vi "FINAL_PROJECT.vi"() -> ()   [LabVIEW 2014]
panel:
  in  "Blank Button 8":bool caption="Blank Button"
  in  "Blank Button 7":bool caption="Blank Button"
  in  "Blank Button 6":bool caption="Blank Button"
  in  "Blank Button 5":bool caption="Blank Button"
  out "LBV":bool
  out "MBV":bool
  out "HBV":bool
  in  "Blank Button 4":bool caption="Blank Button"
  in  "Blank Button 3":bool caption="Blank Button"
  in  "Blank Button 2":bool caption="Blank Button"
  in  "Blank Button":bool
  out "L":bool
  in  "Air Compressor\nstopped/breakdown":bool
  out "Instrument Air Pressure Gauge (Bar)":dbl(knob) scale=0.0..10.0
  out "H":bool
  out "H":bool
  out "Vibration(mm)":u8(slide) scale=0.0..10.0
  out "GD\n%LEL":u8(slide) scale=0.0..20.0
  out "GD":dbl
  out "Vibration Sensor":dbl
  out "H":bool
  out "High Bank Pressure":u8(slide) scale=0.0..400.0
  out "Medium Bank Pressure":u8(slide) scale=0.0..400.0
  out "Low Bank Pressure":u8(slide) scale=0.0..400.0
  out "Storage Pressure Trend":dbl(graph)
  in  "MB Set-point":dbl
  in  "LB Set-point":dbl
  out "Low Bank Pressure":dbl
  out "MB Trend":dbl(graph) caption="LB Trend"
  out "Medium Bank Pressure":dbl
  out "LB Trend":dbl(graph) caption="MB Trend"
  out "High Bank Pressure":dbl
  out "HB Trend":dbl(graph)
  out "H":bool
  out "L":bool
  in  "Low Stage-3 Temperature (After-Cooler) Set-Point":dbl
  in  "High Stage-3 Temperature (After-Cooler) Set-Point":dbl
  in  "Low Stage-3 Temperature Set-Point":dbl
  in  "High Stage-3 Temperature  Set-Point":dbl
  out "H":bool
  out "L":bool
  in  "Low Stage-3 Pressure  Set-Point":dbl
  in  "High Stage-3 Pressure \nSet-Point":dbl
  out "H":bool
  out "L":bool
  out "3-Stage Pressure":u8(slide) scale=0.0..400.0
  out "3-Stage Temperature (After Cooler)":u8(slide) scale=0.0..250.0
  out "3-Stage Temperature":u8(slide) scale=0.0..250.0
  out "3-Stage Pressure":dbl
  out "3-Stage Temperature (After Cooler)":dbl
  out "3-Stage Temperature":dbl
  out "H":bool
  out "L":bool
  in  "Low Stage-2 Temperature (After-Cooler) Set-Point":dbl
  in  "High Stage-2 Temperature (After-Cooler) Set-Point":dbl
  in  "Low Stage-1 Temperature  Set-Point  2":dbl
  in  "High Stage-2 Temperature  Set-Point":dbl
  out "H":bool
  out "L":bool
  in  "Low Stage-2 Pressure  Set-Point":dbl
  in  "High Stage-2 Pressure          Set-Point":dbl
  out "H":bool
  out "L":bool
  out "2-Stage Pressure":u8(slide) scale=0.0..400.0
  out "2-Stage Temperature (After Cooler)":u8(slide) scale=0.0..250.0
  out "2-Stage Temperature":u8(slide) scale=0.0..250.0
  out "2-Stage Pressure":dbl
  out "2-Stage Temperature (After Cooler)":dbl
  out "2-Stage Temperature":dbl
  in  "Critical Vibration Value":dbl
  in  "Gas Detector %LEL       Set-point":dbl
  out "H":bool
  out "L":bool
  in  "Low Stage-1 Temperature (After-Cooler) Set-Point  2":dbl
  in  "High Stage-1 Temperature (After-Cooler) Set-Point":dbl
  in  "Low Stage-1 Temperature  Set-Point":dbl
  in  "High Stage-1 Temperature  Set-Point":dbl
  out "H":bool
  out "L":bool
  out "MFM Total Kg (Inlet)":dbl format="%#_9g"
  in  "Wire cut":bool
  out "Inlet MFM Total Kg Trend (Kg)":dbl(graph)
  out "Discharge MFM Total Kg Trend (Kg)":dbl(graph)
  out "Inlet MFM Flow Rate Trend (Kg/m2)":dbl(graph)
  out "Discharge MFM Flow Rate Trend (Kg/m2)":dbl(graph)
  out "MFM Flow Rate (Discharge)":dbl
  out "MFM Flow Rate (Inlet)":dbl
  out "MFM Total Kg (Discharge)":dbl format="%#_9g"
  out "Storage Pressure":u8(slide) scale=0.0..400.0
  out "De-pressurizing Diaphram Valve":bool
  out "Suction Valve":bool
  in  "Storage /HB Pressure Set-Point":dbl
  out "CO2 Flooding in Progress":bool
  in  "Fire":bool
  out "Fire Detector-2":bool
  out "Fire Detector-1":bool
  out "ESD":bool
  out "Communication Status":string
  out "Compressor Running Status":string
  in  "Low Stage-1 Pressure  Set-Point":dbl
  in  "High Stage-1 Pressure          Set-Point":dbl
  out "H":bool
  out "L":bool
  out "TT-01":dbl
  out "1-Stage Pressure":u8(slide) scale=0.0..400.0
  out "1-Stage Temperature (After Cooler)":u8(slide) scale=0.0..250.0
  out "1-Stage Temperature":u8(slide) scale=0.0..250.0
  out "PT-11":dbl
  out "1-Stage Temperature (After Cooler)":dbl
  out "TT-11":dbl
  in  "Emergency Shutdown":bool
  out "PT-01":dbl
  out "L":bool
  out "H":bool
  in  "Low Inlet Pressure  Set-Point":dbl
  in  "High Inlet Pressure          Set-Point":dbl
  out "Inlet Temperature":u8(slide) scale=0.0..250.0
  out "Inlet Pressure":u8(slide) scale=0.0..40.0
  # "OPERATING PARAMETERS-PRESSURE (barg)"
  # "Suction MFM"
  # "BV"
  # "Filter"
  # "Cooler"
  # "Suction Valve"
  # "Cooler"
  # "OPERATING PARAMETERS-MASS FLOW"
  # "OPERATING PARAMETERS-TEMPERATURE (degC)"
  # "HBV"
  # "Inlet Stage Operating Parameters"
  # "Stage-I Operating Parameters"
  # "Stage-II Operating Parameters"
  # "Stage-III Operating Parameters"
  # "De-Pressurizing\nDiaphragm\nValve"
  # "OPERATING\nPARAMETERS-VIBRATION\n& GAS LEAK"
  # "MBV"
  # "Cooler"
  # "LBV"
  # "Discharge MFM"
  # "CV"
  # "CONFIGURE SET-POINTS"
  # "FIRE SUPPRESSION SAFETY INTERLOCK"
  # "OPERATING PRESSURE TREND"
  # "OPERATING MASS FLOW TREND"
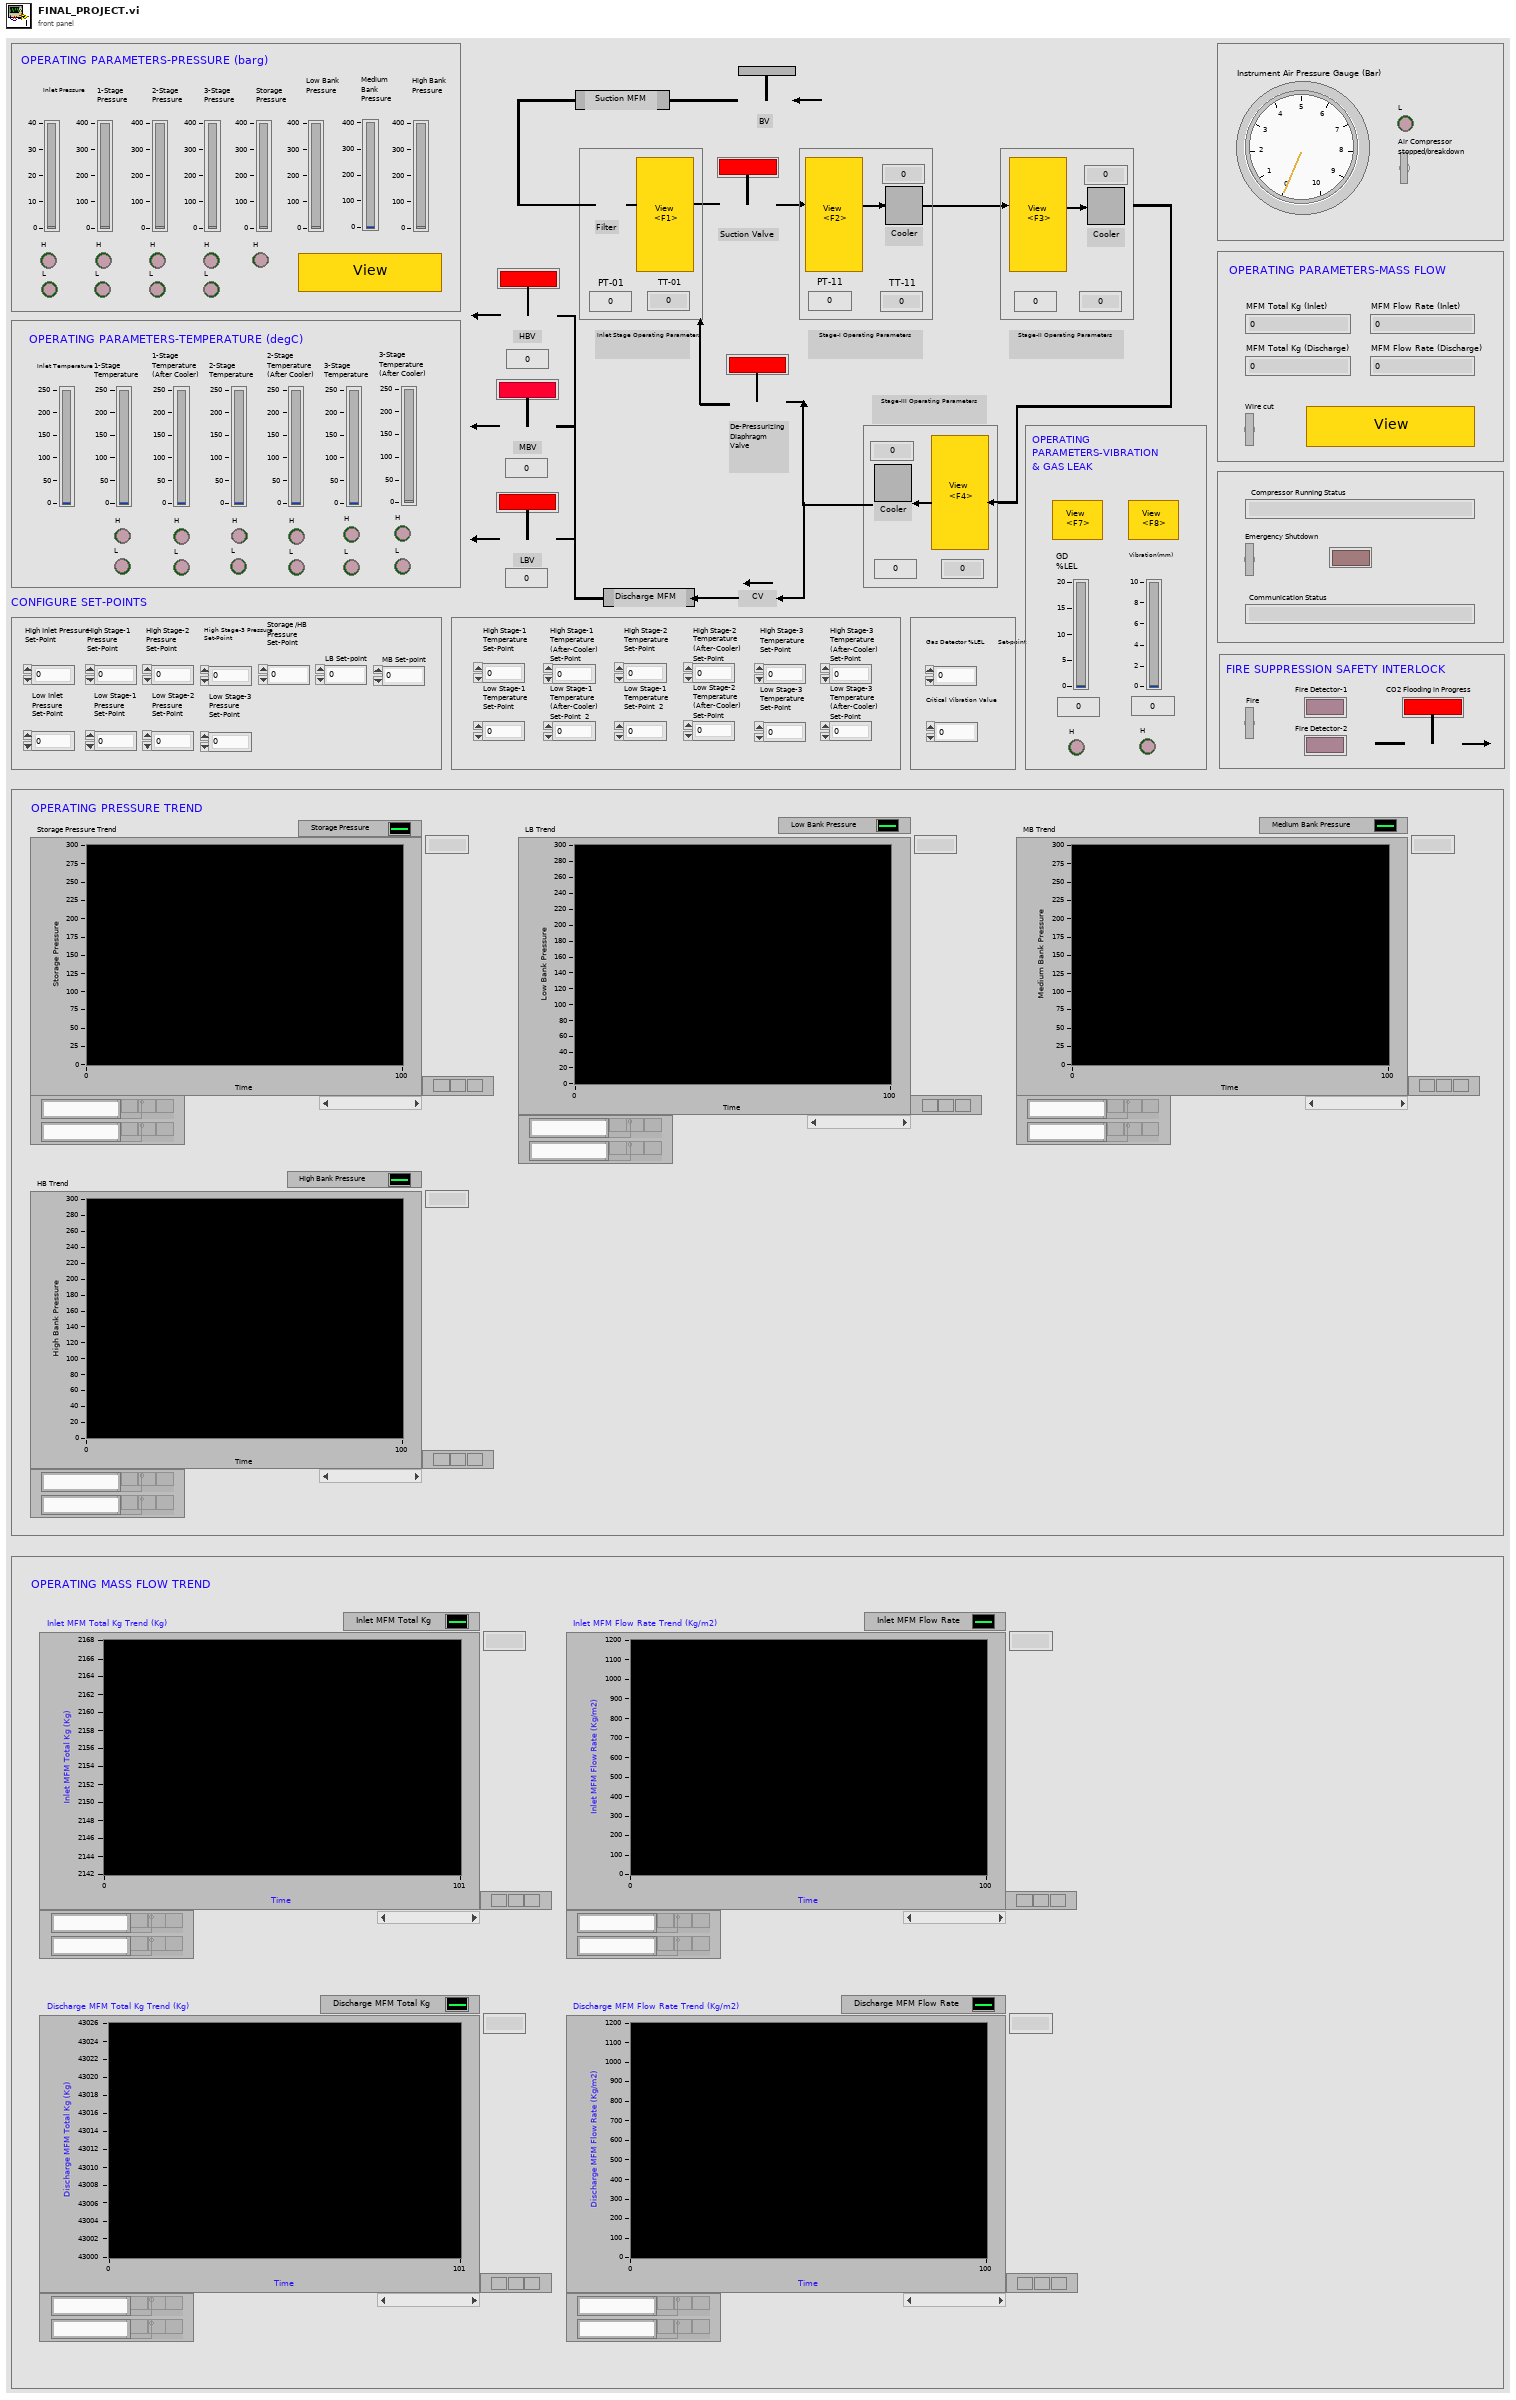
[diagram p1: front panel]
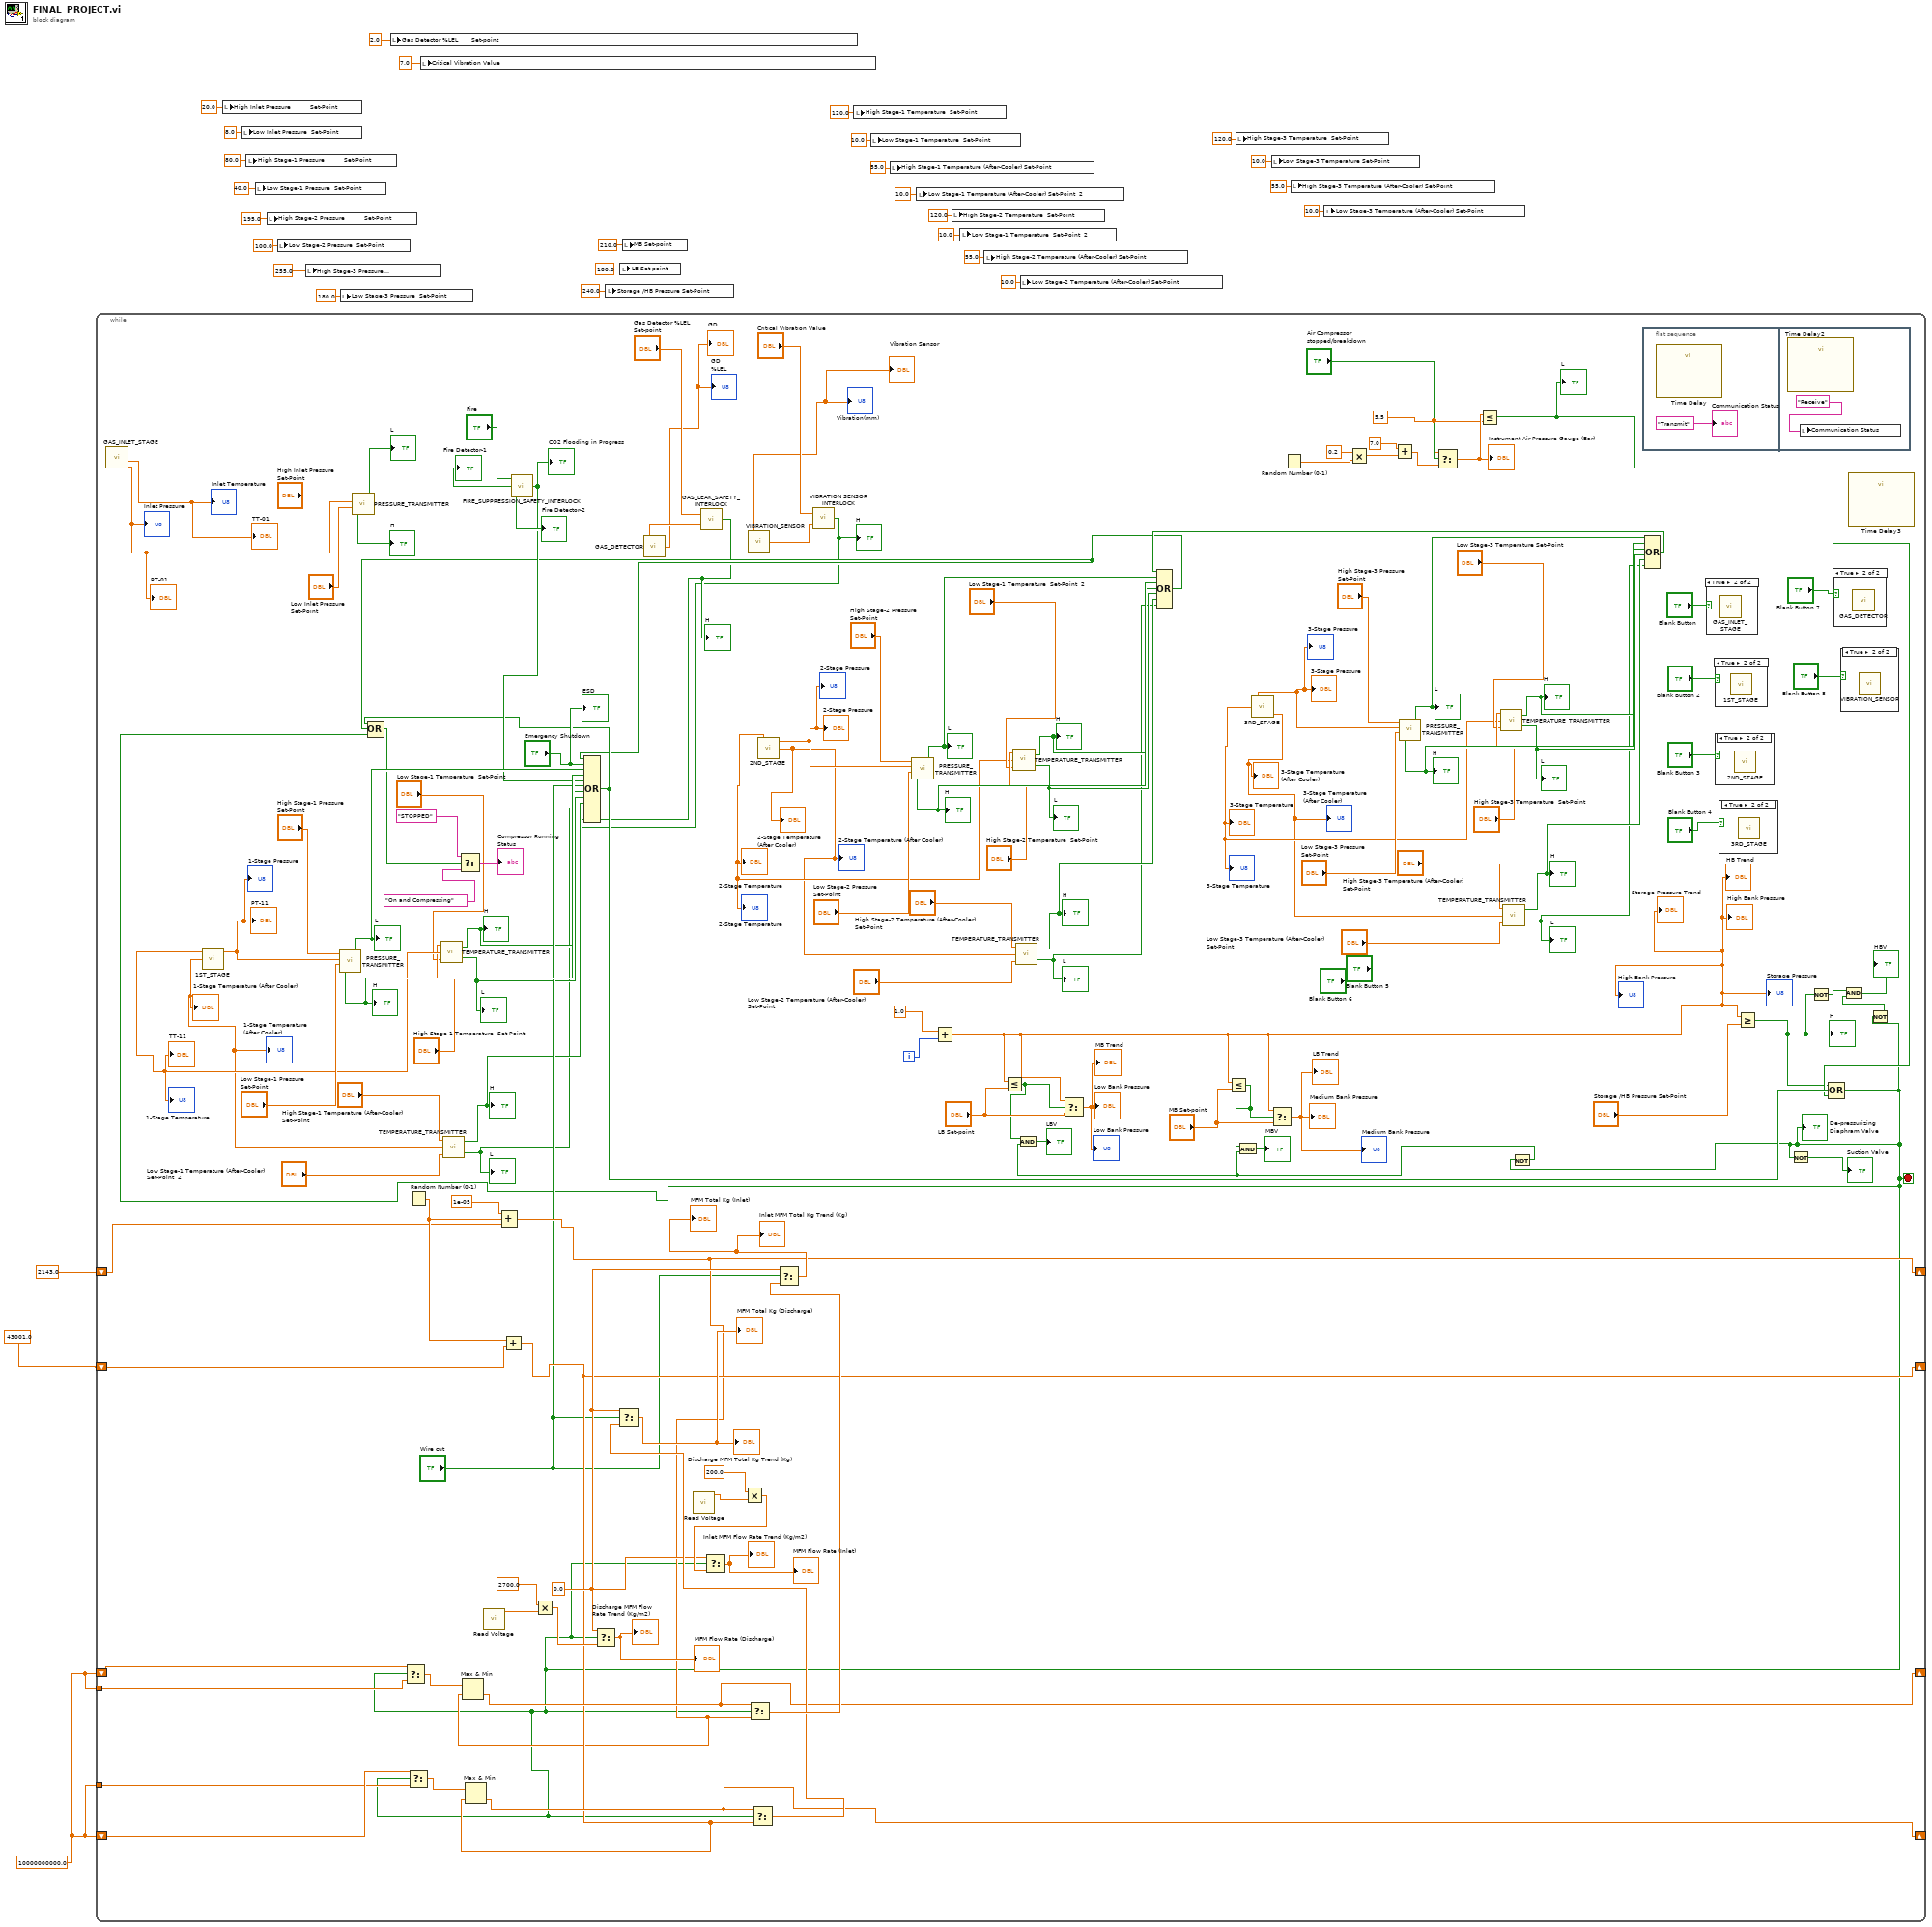
[diagram p0: block diagram]
diagram:
  w26 = 10000000000.0
  n1 = while {
    shift-right: [w118] -> _
    shift-left: 2143.0 -> [w117]
    shift-right: [w119] -> _
    shift-left: 43001.0 -> [w116]
    shift-right: [w120] -> _
    shift-left: w26 -> [w113]
    shift-right: [w121] -> _
    shift-left: w26 -> [w122]
    tunnel: w26 -> [w114]
    tunnel: w26 -> [w112]
    i -> [w142]
    stop <- w35 stop-if-true
    w49 = 5.5
    w123 = 0.0
    n2 = call "GAS_INLET_STAGE.vi"() -> ("Inlet Pressure"=w157:dbl, "Inlet Temperature"=→"Inlet Temperature" →"TT-01":dbl)  [unwired: 2 out]
    "Inlet Pressure" <- w157
    "PT-01" <- w157
    n3 = call "1ST_STAGE.vi"() -> ("Stage-I Pressure Transmitter"=w153:dbl, "Stage 1 Coolant Temperature"=w106:dbl, "Stage-I Temperature Transmitter"=w111:dbl)  [unwired: 3 out]
    "TT-11" <- w111
    "1-Stage Temperature (After Cooler)" <- w106
    "PT-11" <- w153
    "1-Stage Temperature" <- w111
    "1-Stage Temperature (After Cooler)" <- w106
    "1-Stage Pressure" <- w153
    n4 = call "PRESSURE_TRANSMITTER.vi"("Low Value Set-point"="Low Stage-1 Pressure  Set-Point", "Input"=w153, "High Value Set-point"="High Stage-1 Pressure          Set-Point") -> ("Low Limit"=w152:bool, "High Limit"=w148:bool)
    "L" <- w152
    "H" <- w148
    n5 = call "PRESSURE_TRANSMITTER.vi"("Low Value Set-point"="Low Inlet Pressure  Set-Point", "Input"=w157, "High Value Set-point"="High Inlet Pressure          Set-Point") -> ("Low Limit"=→"L":bool, "High Limit"=→"H":bool)
    n6 = Random Number (0-1)() -> (number: 0 to 1=w139:dbl)
    n7 = call "TEMPERATURE_TRANSMITTER.vi"("Lower setpoint"="Low Stage-1 Temperature  Set-Point", "Input"=w111, "Higher setpoint"="High Stage-1 Temperature  Set-Point") -> ("LOW"=w107:bool, "HIGH"=w108:bool)
    "L" <- w107
    "H" <- w108
    n8 = call "TEMPERATURE_TRANSMITTER.vi"("Lower setpoint"="Low Stage-1 Temperature (After-Cooler) Set-Point  2", "Input"=w106, "Higher setpoint"="High Stage-1 Temperature (After-Cooler) Set-Point") -> ("LOW"=w102:bool, "HIGH"=w103:bool)
    "L" <- w102
    "H" <- w103
    n9 = call "Read Voltage.vi"() -> ("voltage"=w134:dbl)  [unwired: 6 in, 1 out]
    n10 = Compound Arithmetic op=ADD(1e-05, w139, w117) -> (w118:dbl)
    n11 = Add(x=w139, y=w116) -> (x+y=w119:dbl)
    n12 = call "FIRE_SUPPRESSION_SAFETY_INTERLOCK.vi"("Fire"="Fire") -> ("CO2 Flooding in Progress"=w143:bool, "Fire Detector-2"=→"Fire Detector-2":bool, "Fire Detector-1"=→"Fire Detector-1":bool)
    "CO2 Flooding in Progress" <- w143
    n13 = Multiply(x=2700.0, y=w134) -> (x*y=w131:dbl)
    n14 = call "GAS_DETECTOR.vi"() -> ("Gas Detector"=→"GD" →"GD\n%LEL":dbl, "Gas Leak (%LEL)"=w65:dbl)
    n15 = call "Read Voltage.vi"() -> ("voltage"=w136:dbl)  [unwired: 6 in, 1 out]
    n16 = call "GAS_LEAK_SAFETY_INTERLOCK.vi"("%LEL"=w65, "%LEL Set-point"="Gas Detector %LEL       Set-point") -> ("Alarm"=w47:bool)
    "H" <- w47
    n17 = Multiply(x=200.0, y=w136) -> (x*y=w130:dbl)
    n18 = call "VIBRATION_SENSOR.vi"() -> ("Vibration (mm)"=w66:dbl, "Vibration Sensor"=→"Vibration Sensor" →"Vibration(mm)":dbl)
    n19 = call "2ND_STAGE.vi"() -> ("Stage-II Temperature Transmitter (After Cooler)"=w59:dbl, "Stage-II Pressure Transmitter"=w70:dbl, "Stage-II Temperature Transmitter"=w71:dbl)  [unwired: 3 out]
    "2-Stage Temperature" <- w71
    "2-Stage Temperature (After Cooler)" <- w59
    "2-Stage Pressure" <- w70
    "2-Stage Temperature" <- w71
    "2-Stage Temperature (After Cooler)" <- w59
    "2-Stage Pressure" <- w70
    n20 = call "VIBRATION SENSOR INTERLOCK.vi"("Operating Vibration Value"=w66, "Critical Vibration Value"="Critical Vibration Value") -> ("Alarm"=w46:bool)
    "H" <- w46
    n21 = call "PRESSURE_TRANSMITTER.vi"("Low Value Set-point"="Low Stage-2 Pressure  Set-Point", "Input"=w70, "High Value Set-point"="High Stage-2 Pressure          Set-Point") -> ("Low Limit"=w97:bool, "High Limit"=w96:bool)
    "L" <- w97
    "H" <- w96
    n22 = Add(x=1.0, y=w142) -> (x+y=w60:dbl)
    "Storage Pressure" <- w60
    "High Bank Pressure" <- w60
    "HB Trend" <- w60
    "Storage Pressure Trend" <- w60
    "High Bank Pressure" <- w60
    n23 = Less Or Equal?(x=w60, y="LB Set-point") -> (x <= y?=w40:bool)
    n24 = call "TEMPERATURE_TRANSMITTER.vi"("Lower setpoint"="Low Stage-1 Temperature  Set-Point  2", "Input"=w71, "Higher setpoint"="High Stage-2 Temperature  Set-Point") -> ("LOW"=w92:bool, "HIGH"=w93:bool)
    "L" <- w92
    "H" <- w93
    n25 = call "TEMPERATURE_TRANSMITTER.vi"("Lower setpoint"="Low Stage-2 Temperature (After-Cooler) Set-Point", "Input"=w59, "Higher setpoint"="High Stage-2 Temperature (After-Cooler) Set-Point") -> ("LOW"=w88:bool, "HIGH"=w89:bool)
    "L" <- w88
    "H" <- w89
    n26 = Select(t=w60, s=w40, f="LB Set-point") -> (s? t:f=→"Low Bank Pressure" →"MB Trend" →"Low Bank Pressure":dbl)
    n27 = Less Or Equal?(x=w60, y="MB Set-point") -> (x <= y?=w43:bool)
    n28 = call "3RD_STAGE.vi"() -> ("Stage 3 Coolant Temperature"=w67:dbl, "Stage-III Temperature Transmitter"=w69:dbl, "Stage-III Pressure Transmitter"=w68:dbl)  [unwired: 3 out]
    "3-Stage Temperature" <- w69
    "3-Stage Temperature (After Cooler)" <- w67
    "3-Stage Pressure" <- w68
    "3-Stage Temperature" <- w69
    "3-Stage Temperature (After Cooler)" <- w67
    "3-Stage Pressure" <- w68
    n29 = Select(t=w60, s=w43, f="MB Set-point") -> (s? t:f=→"Medium Bank Pressure" →"LB Trend" →"Medium Bank Pressure":dbl)
    n30 = Random Number (0-1)() -> (number: 0 to 1=w56:dbl)
    n31 = Multiply(x=0.2, y=w56) -> (x*y=w54:dbl)
    n32 = Add(x=7.0, y=w54) -> (x+y=w51:dbl)
    n33 = call "PRESSURE_TRANSMITTER.vi"("Low Value Set-point"="Low Stage-3 Pressure  Set-Point", "Input"=w68, "High Value Set-point"="High Stage-3 Pressure \nSet-Point") -> ("Low Limit"=w85:bool, "High Limit"=w84:bool)
    "L" <- w85
    "H" <- w84
    n34 = Select(t=w49, s="Air Compressor\nstopped/breakdown", f=w51) -> (s? t:f=w50:dbl)
    "Instrument Air Pressure Gauge (Bar)" <- w50
    n35 = Less Or Equal?(x=w50, y=w49) -> (x <= y?=w48:bool)
    "L" <- w48
    n36 = call "TEMPERATURE_TRANSMITTER.vi"("Lower setpoint"="Low Stage-3 Temperature Set-Point", "Input"=w69, "Higher setpoint"="High Stage-3 Temperature  Set-Point") -> ("LOW"=w80:bool, "HIGH"=w81:bool)
    "L" <- w80
    "H" <- w81
    n37 = call "TEMPERATURE_TRANSMITTER.vi"("Lower setpoint"="Low Stage-3 Temperature (After-Cooler) Set-Point", "Input"=w67, "Higher setpoint"="High Stage-3 Temperature (After-Cooler) Set-Point") -> ("LOW"=w76:bool, "HIGH"=w77:bool)
    "L" <- w76
    "H" <- w77
    n38 = flat-sequence {
      frame #0 {
        n39 = call "Time Delay"() -> ()  [unwired: 11 in, 1 out]
        "Communication Status" <- "Transmit"
      }
      frame #1 {
        n40 = call "Time Delay2"() -> ()  [unwired: 11 in, 1 out]
        n41 = local write "Communication Status"("Receive") -> ()
      }
    }
    n42 = Compound Arithmetic op=OR(w85, w84, w81, w80, w77, w76) -> (w75:bool)
    n43 = Compound Arithmetic op=OR(w75, w97, w96, w93, w92, w89, w88) -> (w72:bool)
    n44 = Compound Arithmetic op=OR(w72, "Emergency Shutdown", w152, w148, w143, "Wire cut", w108, w107, w103, w102, w47, w46) -> (w73:bool)
    n45 = case shown="True" "Blank Button" {
      frame False {
      }
      frame True {
        n46 = call "GAS_INLET_STAGE.vi"() -> ()  [unwired: 4 out]
      }
    }
    n47 = case shown="True" "Blank Button 2" {
      frame False {
      }
      frame True {
        n48 = call "1ST_STAGE.vi"() -> ()  [unwired: 6 out]
      }
    }
    n49 = case shown="True" "Blank Button 3" {
      frame False {
      }
      frame True {
        n50 = call "2ND_STAGE.vi"() -> ()  [unwired: 6 out]
      }
    }
    n51 = case shown="True" "Blank Button 4" {
      frame False {
      }
      frame True {
        n52 = call "3RD_STAGE.vi"() -> ()  [unwired: 6 out]
      }
    }
    n53 = Greater Or Equal?(x=w60, y="Storage /HB Pressure Set-Point") -> (x >= y?=w36:bool)
    "H" <- w36
    n54 = Not(x=w36) -> (.not. x?=w37:bool)
    n55 = Compound Arithmetic op=OR(w36, w73, w48) -> (w35:bool)
    "De-pressurizing Diaphram Valve" <- w35
    n56 = Compound Arithmetic op=OR(w73, w72, w35) -> (w74:bool)
    n57 = Select(t=w113, s=w35, f=w112) -> (s? t:f=w133:dbl)
    n58 = Select(t=w122, s=w35, f=w114) -> (s? t:f=w132:dbl)
    n59 = Select(t="STOPPED", s=w74, f="On and Compressing") -> (s? t:f=→"Compressor Running Status":string)
    n60 = Max & Min(x=w133, y=w118) -> (min(x,y)=w120:dbl)  [unwired: 1 out]
    n61 = Max & Min(x=w132, y=w119) -> (min(x,y)=w121:dbl)  [unwired: 1 out]
    n62 = Select(t=w123, s=w35, f=w131) -> (s? t:f=→"Discharge MFM Flow Rate Trend (Kg/m2)" →"MFM Flow Rate (Discharge)":dbl)
    n63 = Select(t=w123, s=w35, f=w130) -> (s? t:f=→"Inlet MFM Flow Rate Trend (Kg/m2)" →"MFM Flow Rate (Inlet)":dbl)
    n64 = Select(t=w120, s=w35, f=w118) -> (s? t:f=w126:dbl)
    n65 = Select(t=w121, s=w35, f=w119) -> (s? t:f=w125:dbl)
    n66 = Select(t=w123, s="Wire cut", f=w125) -> (s? t:f=→"Discharge MFM Total Kg Trend (Kg)" →"MFM Total Kg (Discharge)":dbl)
    n67 = Select(t=w123, s="Wire cut", f=w126) -> (s? t:f=→"MFM Total Kg (Inlet)" →"Inlet MFM Total Kg Trend (Kg)":dbl)
    n68 = Not(x=w35) -> (.not. x?=w39:bool)
    n69 = And(x=w40, y=w39) -> (x .and. y?=→"LBV":bool)
    n70 = And(x=w43, y=w39) -> (x .and. y?=→"MBV":bool)
    n71 = Not(x=w35) -> (.not. x?=→"Suction Valve":bool)
    n72 = case shown="True" "Blank Button 7" {
      frame False {
      }
      frame True {
        n73 = call "GAS_DETECTOR.vi"() -> ()  [unwired: 2 out]
      }
    }
    n74 = case shown="True" "Blank Button 8" {
      frame False {
      }
      frame True {
        n75 = call "VIBRATION_SENSOR.vi"() -> ()  [unwired: 2 out]
      }
    }
    n76 = call "Time Delay3"() -> ()  [unwired: 11 in, 1 out]
    n77 = Not(x=w35) -> (.not. x?=w34:bool)
    n78 = And(x=w37, y=w34) -> (x .and. y?=→"HBV":bool)
    "ESD" <- "Emergency Shutdown"
  }
  n79 = local write "High Inlet Pressure          Set-Point"(20.0 ("High Inlet Pressure          Set-Point")) -> ()
  n80 = local write "Low Inlet Pressure  Set-Point"(8.0 ("Low Inlet Pressure  Set-Point")) -> ()
  n81 = local write "High Stage-1 Pressure          Set-Point"(80.0 ("High Stage-1 Pressure          Set-Point")) -> ()
  n82 = local write "Low Stage-1 Pressure  Set-Point"(40.0 ("Low Stage-1 Pressure  Set-Point")) -> ()
  n83 = local write "High Stage-2 Pressure          Set-Point"(195.0 ("High Stage-2 Pressure          Set-Point")) -> ()
  n84 = local write "Low Stage-2 Pressure  Set-Point"(100.0 ("Low Stage-2 Pressure  Set-Point")) -> ()
  n85 = local write "High Stage-3 Pressure \nSet-Point"(255.0 ("High Stage-3 Pressure          Set-Point")) -> ()
  n86 = local write "Low Stage-3 Pressure  Set-Point"(180.0 ("Low Stage-3 Pressure  Set-Point")) -> ()
  n87 = local write "Gas Detector %LEL       Set-point"(2.0 ("Gas Detector %LEL       Set-point")) -> ()
  n88 = local write "Critical Vibration Value"(7.0 ("Critical Vibration Value")) -> ()
  n89 = local write "Storage /HB Pressure Set-Point"(240.0 ("Storage /HB Pressure Set-Point")) -> ()
  n90 = local write "LB Set-point"(180.0 ("LB Set-point")) -> ()
  n91 = local write "MB Set-point"(210.0 ("MB Set-point")) -> ()
  n92 = local write "High Stage-1 Temperature  Set-Point"(120.0 ("High Stage-1 Temperature  Set-Point")) -> ()
  n93 = local write "Low Stage-1 Temperature  Set-Point"(10.0 ("Low Stage-1 Temperature  Set-Point")) -> ()
  n94 = local write "High Stage-1 Temperature (After-Cooler) Set-Point"(55.0 ("High Stage-1 Temperature (After-Cooler) Set-Point")) -> ()
  n95 = local write "Low Stage-1 Temperature (After-Cooler) Set-Point  2"(10.0 ("Low Stage-1 Temperature (After-Cooler) Set-Point  2")) -> ()
  n96 = local write "High Stage-2 Temperature  Set-Point"(120.0 ("High Stage-2 Temperature  Set-Point")) -> ()
  n97 = local write "Low Stage-1 Temperature  Set-Point  2"(10.0 ("Low Stage-1 Temperature  Set-Point  2")) -> ()
  n98 = local write "High Stage-2 Temperature (After-Cooler) Set-Point"(55.0 ("High Stage-2 Temperature (After-Cooler) Set-Point")) -> ()
  n99 = local write "Low Stage-2 Temperature (After-Cooler) Set-Point"(10.0 ("Low Stage-2 Temperature (After-Cooler) Set-Point")) -> ()
  n100 = local write "High Stage-3 Temperature  Set-Point"(120.0 ("High Stage-3 Temperature  Set-Point")) -> ()
  n101 = local write "Low Stage-3 Temperature Set-Point"(10.0 ("Low Stage-3 Temperature Set-Point")) -> ()
  n102 = local write "High Stage-3 Temperature (After-Cooler) Set-Point"(55.0 ("High Stage-3 Temperature (After-Cooler) Set-Point")) -> ()
  n103 = local write "Low Stage-3 Temperature (After-Cooler) Set-Point"(10.0 ("Low Stage-3 Temperature (After-Cooler) Set-Point")) -> ()
